vi "New Basic Scope.vi"   [LabVIEW 2018, in "GLog.lvlib" / "Basic.lvclass"]
uses:
  Basic.lvclass
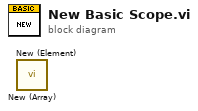
[diagram p0: block diagram]
diagram:
  n1 = call "New (Array).vi"() -> ()  [unwired: 11 in, 1 out]
  n2 = call "New (Element).vi"() -> ()  [unwired: 11 in, 1 out]
